vi "2019-05-09_shift_register_gaus_sum.vi"() -> ()   [LabVIEW 2018]
panel:
  out "숫자형 컨트롤":i32
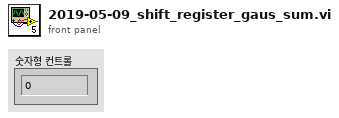
[diagram p1: front panel]
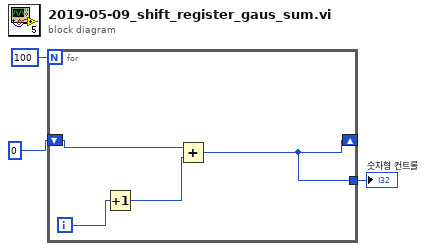
[diagram p0: block diagram]
diagram:
  n1 = for {
    N: 100 -> [_]
    shift-right: [w4] -> _
    shift-left: 0 -> [w5]
    tunnel: [w4] -> w1
    i -> [w7]
    n2 = Increment(x=w7) -> (x+1=w6:i32)
    n3 = Add(x=w5, y=w6) -> (x+y=w4:i32)
  }
  "숫자형 컨트롤" <- w1
